vi "luaL_loadfile.vi"(8 "error in (no error)":errorcluster, 10 "filename":path, 11 "lua_state_p":u64) -> (0 "error out":errorcluster, 3 "lua_state_p out":u64)   [LabVIEW 2020, in "lua.dll.lvlib"]
uses:
  lua.dll.lvlib
  lua54.dll
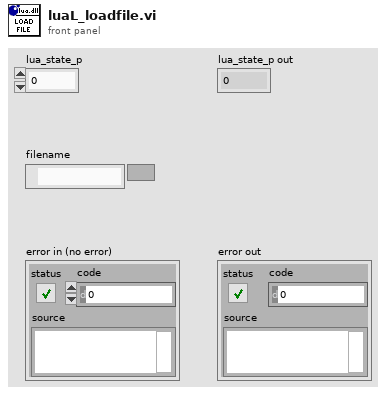
[diagram p1: front panel]
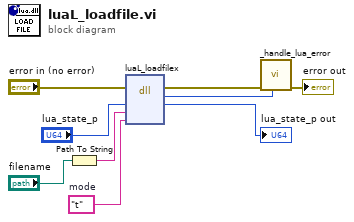
[diagram p0: block diagram]
diagram:
  w4 = "t"  # mode
  n1 = Path To String(path="filename") -> (string=w5:string)
  n2 = dll-call lib="C:/Users/Nicholas Folse/Documents/workspace/github-tauterra.llc/Lua for LabVIEW/lib/lua.dll/lua54**.*" fn="luaL_loadfilex"(error in="error in (no error)", "lua_state_p"="lua_state_p", "filename"=w5, "mode"=w4) -> (error out=w3:errorcluster, "errcode"=w1:i32, "lua_state_p"=→"lua_state_p out":u64)  [unwired: 4 in, 1 out]
  n3 = call "_handle_lua_error.vi"("lua status"=w1, "error in (no error)"=w3) -> ("error out"=→"error out":errorcluster)  [unwired: 9 in]
